vi "ql2proto_term_type_encode.vi"(11 "term_type":T1) -> (2 "term_type_ids":u32[](array[numeric])=[1, 2, 3, 10, 11, 169, 153, 12, 13, 14, 15, 16, 78, 17, 18, 19, 20, 21, 22, 23, 24, 25, 26, 27, 28, 183, 184, 185, 29, 80, 95, 88, 89, 90, 91, 30, 70, 71, 87, 93, 31, 94, 186, 143, 32, 96, 33, 34, 35, 36, 182, 37, 38, 187, 39, 40, 41, 42, 43, 86, 44, 45, 170, 48, 49, 50, 72, 173, 82, 83, 84, 85, 51, 52, 53, 54, 55, 56, 57, 58, 59, 60, 61, 62, 174, 175, 177, 176, 179, 138, 188, 75, 76, 77, 139, 140, 156, 189, 190, 64, 65, 66, 67, 68, 69, 73, 74, 79, 97, 141, 142, 81, 92, 98, 99, 100, 101, 102, 103, 104, 105, 106, 126, 127, 128, 129, 130, 131, 132, 133, 134, 135, 136, 107, 108, 109, 110, 111, 112, 113, 114, 115, 116, 117, 118, 119, 120, 121, 122, 123, 124, 125, 137, 144, 145, 146, 147, 148, 149, 150, 151, 152, 154, 155, 157, 158, 159, 160, 161, 162, 163, 164, 165, 166, 167, 168, 171, 172, 180, 181, 191, 192, 193, 194, 195, 196], 3 "id":u32)   [LabVIEW 2017]
uses:
  ql2proto_term_type.ctl
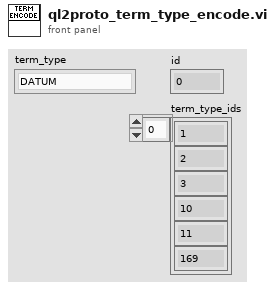
[diagram p1: front panel]
types:
  T1 = typedef "ql2proto_term_type.ctl" = enum8{"DATUM", "MAKE_ARRAY", "MAKE_OBJ", "VAR", "JAVASCRIPT", "UUID", "HTTP", "ERROR", "IMPLICIT_VAR", "DB", "TABLE", "GET", "GET_ALL", "EQ", "NE", "LT", "LE", "GT", "GE", "NOT", "ADD", "SUB", "MUL", "DIV", "MOD", "FLOOR", "CEIL", "ROUND", "APPEND", "PREPEND", "DIFFERENCE", "SET_INSERT", "SET_INTERSECTION", "SET_UNION", "SET_DIFFERENCE", "SLICE", "SKIP", "LIMIT", "OFFSETS_OF", "CONTAINS", "GET_FIELD", "KEYS", "VALUES", "OBJECT", "HAS_FIELDS", "WITH_FIELDS", "PLUCK", "WITHOUT", "MERGE", "BETWEEN_DEPRECATED", "BETWEEN", "REDUCE", "MAP", "FOLD", "FILTER", "CONCAT_MAP", "ORDER_BY", "DISTINCT", "COUNT", "IS_EMPTY", "UNION", "NTH", "BRACKET", "INNER_JOIN", "OUTER_JOIN", "EQ_JOIN", "ZIP", "RANGE", "INSERT_AT", "DELETE_AT", "CHANGE_AT", "SPLICE_AT", "COERCE_TO", "TYPE_OF", "UPDATE", "DELETE", "REPLACE", "INSERT", "DB_CREATE", "DB_DROP", "DB_LIST", "TABLE_CREATE", "TABLE_DROP", "TABLE_LIST", "CONFIG", "STATUS", "WAIT", "RECONFIGURE", "REBALANCE", "SYNC", "GRANT", "INDEX_CREATE", "INDEX_DROP", "INDEX_LIST", "INDEX_STATUS", "INDEX_WAIT", "INDEX_RENAME", "SET_WRITE_HOOK", "GET_WRITE_HOOK", "FUNCALL", "BRANCH", "OR", "AND", "FOR_EACH", "FUNC", "ASC", "DESC", "INFO", "MATCH", "UPCASE", "DOWNCASE", "SAMPLE", "DEFAULT", "JSON", "ISO8601", "TO_ISO8601", "EPOCH_TIME", "TO_EPOCH_TIME", "NOW", "IN_TIMEZONE", "DURING", "DATE", "TIME_OF_DAY", "TIMEZONE", "YEAR", "MONTH", "DAY", "DAY_OF_WEEK", "DAY_OF_YEAR", "HOURS", "MINUTES", "SECONDS", "TIME", "MONDAY", "TUESDAY", "WEDNESDAY", "THURSDAY", "FRIDAY", "SATURDAY", "SUNDAY", "JANUARY", "FEBRUARY", "MARCH", "APRIL", "MAY", "JUNE", "JULY", "AUGUST", "SEPTEMBER", "OCTOBER", "NOVEMBER", "DECEMBER", "LITERAL", "GROUP", "SUM", "AVG", "MIN", "MAX", "SPLIT", "UNGROUP", "RANDOM", "CHANGES", "ARGS", "BINARY", "GEOJSON", "TO_GEOJSON", "POINT", "LINE", "POLYGON", "DISTANCE", "INTERSECTS", "INCLUDES", "CIRCLE", "GET_INTERSECTING", "FILL", "GET_NEAREST", "POLYGON_SUB", "TO_JSON_STRING", "MINVAL", "MAXVAL", "BIT_AND", "BIT_OR", "BIT_XOR", "BIT_NOT", "BIT_SAL", "BIT_SAR", "invalid"}
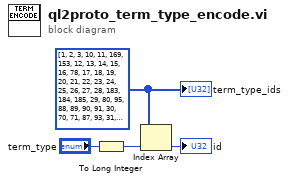
[diagram p0: block diagram]
diagram:
  w4 = u32[] [1, 2, 3, 10, 11, 169, 153, 12, 13, 14, 15, 16, 78, 17, 18, 19, 20, 21, 22, 23, 24, 25, 26, 27, 28, 183, 184, 185, 29, 80, 95, 88, 89, 90, 91, 30, 70, 71, 87, 93, 31, 94, 186, 143, 32, 96, 33, 34, 35, 36, 182, 37, 38, 187, 39, 40, 41, 42, 43, 86, 44, 45, 170, 48, 49, 50, 72, 173, 82, 83, 84, 85, 51, 52, 53, 54, 55, 56, 57, 58, 59, 60, 61, 62, 174, 175, 177, 176, 179, 138, 188, 75, 76, 77, 139, 140, 156, 189, 190, 64, 65, 66, 67, 68, 69, 73, 74, 79, 97, 141, 142, 81, 92, 98, 99, 100, 101, 102, 103, 104, 105, 106, 126, 127, 128, 129, 130, 131, 132, 133, 134, 135, 136, 107, 108, 109, 110, 111, 112, 113, 114, 115, 116, 117, 118, 119, 120, 121, 122, 123, 124, 125, 137, 144, 145, 146, 147, 148, 149, 150, 151, 152, 154, 155, 157, 158, 159, 160, 161, 162, 163, 164, 165, 166, 167, 168, 171, 172, 180, 181, 191, 192, 193, 194, 195, 196] ("ids")
  n1 = To Long Integer(number="term_type") -> (32bit integer=w2:i32)
  n2 = Index Array(array=w4, index=w2) -> (element=→"id":u32)
  "term_type_ids" <- w4
